vi "Read Panel Layout from VI.vi"(8 "error in":errorcluster, 11 "VI refnum":refnum<vi>) -> (0 "error out":errorcluster, 3 "panel layout out":refnum<class "VI Panel Layout.lvclass">)   [LabVIEW 2012, in "NI_SE_Front Panel Layout.lvlib" / "VI Panel Layout.lvclass"]
doc: "Create a panel layout description from an existing VI. Every object on the front panel of the VI will be added to the panel layout description."
uses:
  VI Panel Layout.lvclass
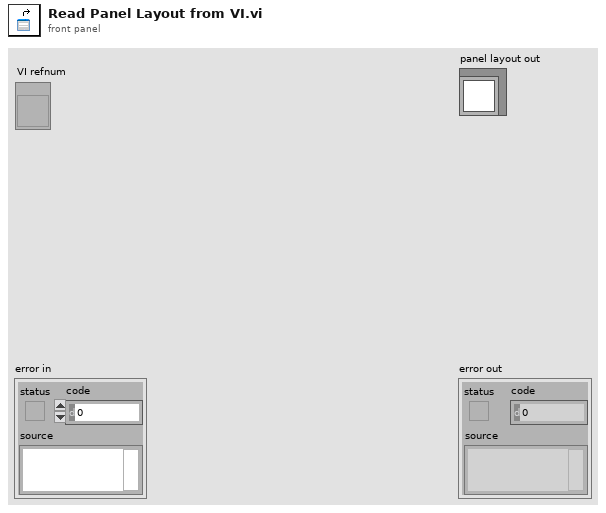
[diagram p1: front panel]
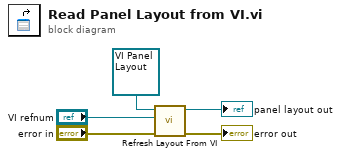
[diagram p0: block diagram]
diagram:
  n1 = call "Refresh Layout From VI.vi"("error in"="error in", "VI refnum"="VI refnum", "VI Panel Layout in"=refnum<class "VI Panel Layout.lvclass"> refnum ("VI Panel Layout out")) -> ("error out"=→"error out":errorcluster, "VI Panel Layout out"=→"panel layout out":refnum<class "VI Panel Layout.lvclass">)  [unwired: 5 in, 2 out]
